vi "Start Tracing.vi"   [LabVIEW 2010, in "NI IO Trace.lvlib"]
doc: "Commands NI I/O Trace to start logging National Instruments API calls. Logs can be stored to file or kept in local memory, depending on the VI instance selected."
uses:
  <vilib>/NiIOTrace/NI IO Trace.lvlib
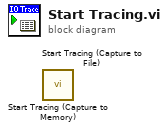
[diagram p0: block diagram]
diagram:
  n1 = call <vilib>:"Start Tracing (Capture to Memory).vi"() -> ()  [unwired: 11 in, 1 out]
  n2 = call <vilib>:"Start Tracing (Capture to File).vi"() -> ()  [unwired: 11 in, 1 out]
